vi "Flatten FIFO Config.vi"(11 "FIFO Config in":T1) -> (3 "Flattened FIFO Config":u8[](array[numeric]))   [LabVIEW 2021, in "ChannelCommon.lvlib"]
uses:
  ChannelCommon.lvlib
  typedef/FIFO Config.ctl
  <vilib>/CIF Foundation/CIF Utilities/DataTypes/DataTypes_CIF_U.lvlib
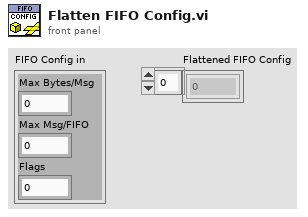
[diagram p1: front panel]
types:
  T1 = typedef "ChannelCommon.lvlib/FIFO Config.ctl" = cluster{"Max Bytes/Msg":u64, "Max Msg/FIFO":u64, "Flags":u64}
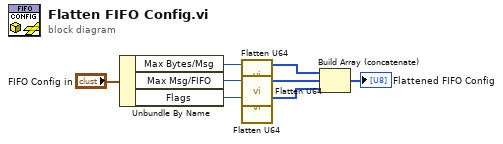
[diagram p0: block diagram]
diagram:
  n1 = Unbundle By Name("FIFO Config in") -> ("Max Bytes/Msg"=w2:u64, "Max Msg/FIFO"=w8:u64, "Flags"=w7:u64)
  n2 = call <vilib>:"Flatten U64.vi"("U64"=w2) -> ("Flat Data"=w1:u8[])  [unwired: 4 in]
  n3 = call <vilib>:"Flatten U64.vi"("U64"=w8) -> ("Flat Data"=w6:u8[])  [unwired: 4 in]
  n4 = call <vilib>:"Flatten U64.vi"("U64"=w7) -> ("Flat Data"=w5:u8[])  [unwired: 4 in]
  n5 = Build Array (concatenate)(w1, w6, w5) -> (→"Flattened FIFO Config":u8[])
